vi "Camera 2020 setup.vi"() -> ()   [LabVIEW 2020]
uses:
  <vilib>/vision/driver/IMAQdx.llb/IMAQdx Camera Control Mode.ctl
  <vilib>/vision/driver/NI_Vision_Acquisition_Software.lvlib
panel:
  out "error out 3":errorcluster
  out "error out 2":errorcluster
  in  "stop":bool
  out "Image":T1(plugin-control)
  out "error out":errorcluster
  in  "Camera Control Mode":T2
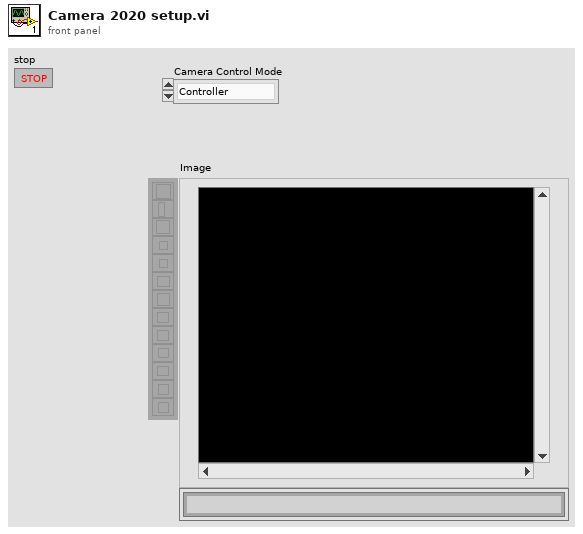
[diagram p1: front panel]
types:
  T1 = typedef "IMAQ Image.ctl" = refnum<image>
  T2 = typedef "NI_Vision_Acquisition_Software.lvlib/IMAQdx Camera Control Mode.ctl" = enum32{"Controller", "Listener"}
  T3 = typedef "IMAQdx.ctl" = refnum<k21>
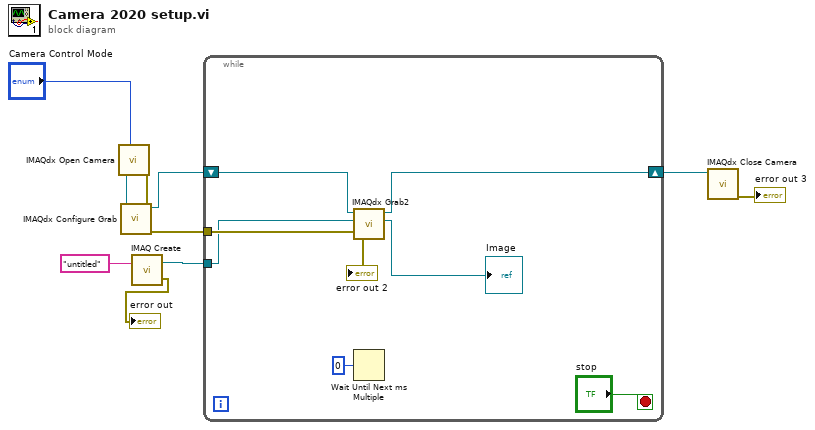
[diagram p0: block diagram]
diagram:
  n1 = call <vilib>:"IMAQdx Open Camera.vi"("Camera Control Mode"="Camera Control Mode") -> ("error out"=w8:errorcluster, "Session Out"=w9:T3)  [unwired: 9 in]
  n2 = call <vilib>:"IMAQdx Configure Grab.vi"("error in"=w8, "Session In"=w9) -> ("error out"=w4:errorcluster, "Session Out"=w7:T3)  [unwired: 8 in]
  n3 = call "IMAQ Create"("Image Name"="untitled") -> ("New Image"=w2:T1, "error out"=→"error out":errorcluster)  [unwired: 4 in]
  n4 = while {
    shift-right: [w16] -> w5
    shift-left: w7 -> [w18]
    tunnel: w4 -> [w14]
    tunnel: w2 -> [w11]
    stop <- "stop" stop-if-true
    n5 = call <vilib>:"IMAQdx Grab2.vi"("error in"=w14, "Image In"=w11, "Session In"=w18) -> ("error out"=→"error out 2":errorcluster, "Image Out"=→"Image":T1, "Session Out"=w16:T3)  [unwired: 5 in, 1 out]
    n6 = Wait Until Next ms Multiple(millisecond multiple=u32 0) -> ()  [unwired: 1 out]
  }
  n7 = call <vilib>:"IMAQdx Close Camera.vi"("Session In"=w5) -> ("error out"=→"error out 3":errorcluster)  [unwired: 10 in]
